vi "PRL TS Clip Array.vi"(6 "Get Full Buffer":bool, 7 "Greater(F)/Greater or Equal(T)":bool, 9 "Window Size":dbl, 10 "Start Timestamp":timestamp, 11 "Timestamp In":timestamp[](array[timestamp])) -> (1 "Index":i32, 2 "Has Data?":bool, 3 "Timestamp Out":timestamp[](array[timestamp]))   [LabVIEW 2013, in "PMU Recorder Light.lvlib"]
doc: "Clips the input timestamp array on a given time, and returns the corresponding buffer index so that the other buffers can be clipped at the same point."
uses:
  PMU Recorder Light.lvlib
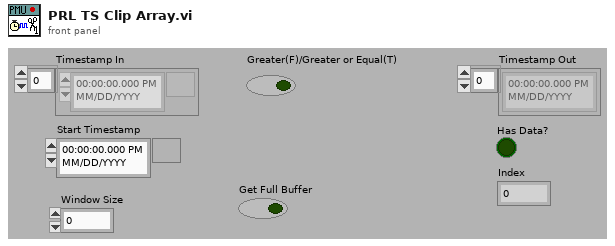
[diagram p1: front panel]
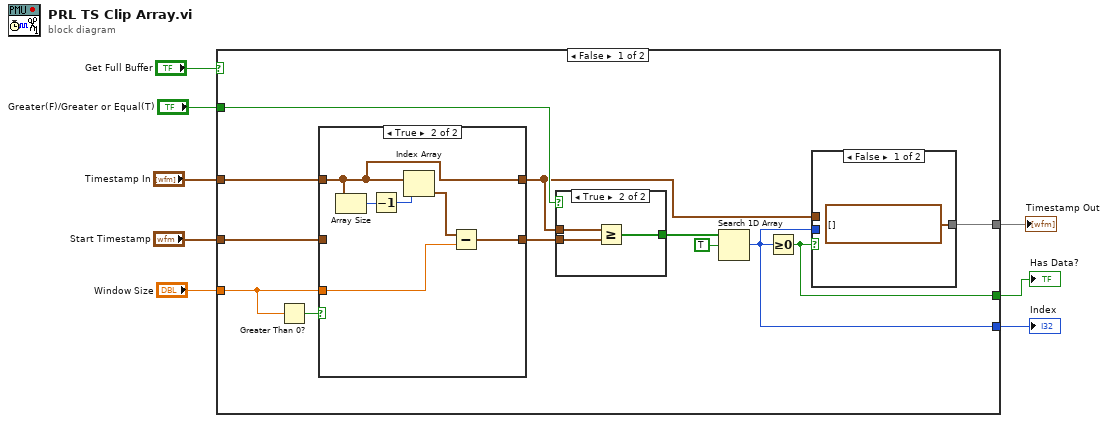
[diagram p0: block diagram]
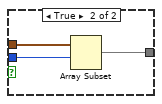
[diagram p3: hidden frame]
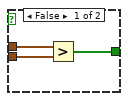
[diagram p4: hidden frame]
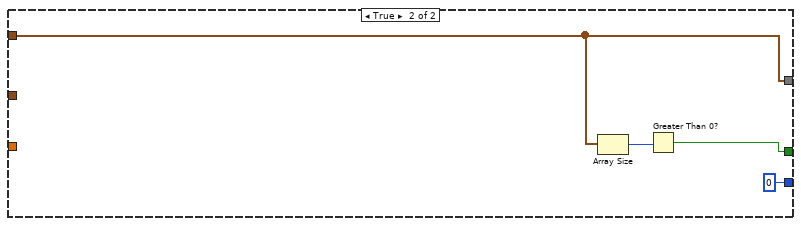
[diagram p5: hidden frame]
diagram:
  n1 = case shown="False" "Get Full Buffer" {
    tunnel: "Greater(F)/Greater or Equal(T)" -> [w20 _]
    tunnel: [w17 w40] -> w7
    tunnel: [w16 0 ("index of element")] -> w6
    tunnel: [w15 w42] -> w5
    tunnel: "Timestamp In" -> [w13 w42]
    tunnel: "Window Size" -> [w12 _]
    tunnel: "Start Timestamp" -> [w11 _]
    frame False {
      n2 = Greater Than 0?(x=w12) -> (x > 0?=w14:bool)
      n3 = case shown="True" w14 {
        tunnel: w13 -> [w22 w23]
        tunnel: w12 -> [_ w25]
        tunnel: w11 -> [w21 _]
        tunnel: [w21 w24] -> w10
        tunnel: [w22 w23] -> w9
        frame False {
        }
        frame True {
          n4 = Array Size(array=w23) -> (size(s)=w28:i32)
          n5 = Decrement(x=w28) -> (x-1=w27:i32)
          n6 = Index Array(array=w23, index=w27) -> (element=w26:timestamp)
          n7 = Subtract(x=w26, y=w25) -> (x-y=w24:timestamp)
        }
      }
      n8 = case shown="True" w20 {
        tunnel: w9 -> [w33 w36]
        tunnel: w10 -> [w35 w38]
        tunnel: [w34 w37] -> w18
        frame False {
          n9 = Greater?(x=w33, y=w35) -> (0:w34:bool[])
        }
        frame True {
          n10 = Greater Or Equal?(x=w36, y=w38) -> (x >= y?=w37:bool[])
        }
      }
      n11 = Search 1D Array(1D array=w18, element=TRUE) -> (index of element=w16:i32)  [unwired: 1 in]
      n12 = Greater Or Equal To 0?(x=w16) -> (x >= 0?=w17:bool)
      n13 = case shown="False" w17 {
        tunnel: w9 -> [_ w32]
        tunnel: w16 -> [_ w31]
        tunnel: [timestamp[] [] w30] -> w15
        frame False {
        }
        frame True {
          n14 = Array Subset(array=w32, index=w31) -> (w30:timestamp[])  [unwired: 1 in]
        }
      }
    }
    frame True {
      n15 = Array Size(array=w42) -> (size(s)=w41:i32)
      n16 = Greater Than 0?(x=w41) -> (x > 0?=w40:bool)
    }
  }
  "Timestamp Out" <- w5
  "Index" <- w6
  "Has Data?" <- w7
